vi "Return Devices with Forecasts.vi"(8 "Bus by ID":T2[](array[typedef]), 9 "ForecastData_Long":variant, 10 "DER_Info":variant, 11 "Generic Optimization in":refnum<class "Generic Optimization.lvclass">) -> (1 "Device Buses":dbl[](array[numeric]), 2 "Forecasts with Devices":T4[](array[typedef]), 3 "dup Generic Optimization out":refnum<class "Generic Optimization.lvclass">, 5 "Devices with Empty Forecasts":T1[](array[typedef]))   [LabVIEW 2018, in "Generic Optimization Actor.lvlib" / "Generic Optimization.lvclass"]
uses:
  Generic Optimization.lvclass
  <vilib>/ORNL/CSEISMIC DDS/CSEISMIC DDS Base/Data Types/ForecastData_Data.ctl
  <vilib>/ORNL/CSEISMIC DDS/CSEISMIC DDS Base/Data Types/Controls/DeviceID.ctl
  <vilib>/ORNL/CSEISMIC DDS/CSEISMIC DDS Base/Data Types/DER_Info.ctl
  Optimization Controls/Bus by ID.ctl
  C:/Users/Administrator/Desktop/2018LabVIEW EMS/EMS Generic Actor/EMS Generic/EMS Generic.lvclass
  <vilib>/ORNL/CSEISMIC DDS/CSEISMIC DDS Base/Data Types/Controls/DeviceClass Selector.ctl
  <vilib>/ORNL/CSEISMIC DDS/CSEISMIC DDS Base/CSEISMIC DDS.lvclass
  EMS Generic Actor/EMS Generic/EMS Generic.lvclass
panel:
  out "Devices with Forecasts":T3[](array[typedef])
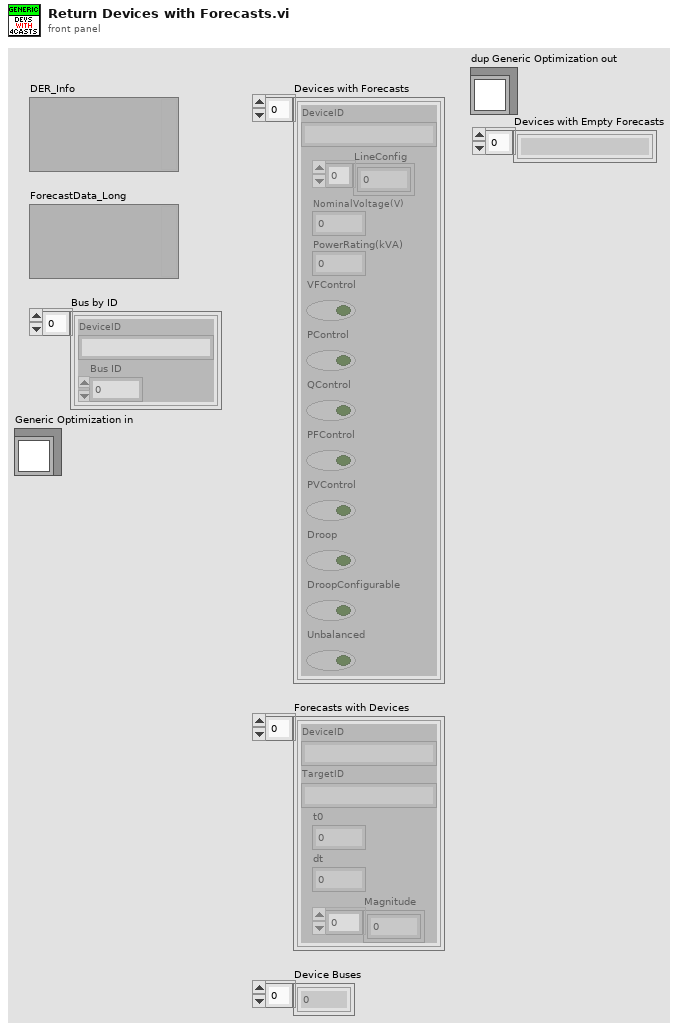
[diagram p1: front panel]
types:
  T1 = typedef "CSEISMIC DDS.lvlib/CSEISMIC DDS.lvclass/DeviceID.ctl" = string
  T2 = typedef "Generic Optimization Actor.lvlib/Generic Optimization.lvclass/Bus by ID.ctl" = cluster{"DeviceID":T1, "Bus ID":dbl}
  T3 = typedef "CSEISMIC DDS.lvlib/CSEISMIC DDS.lvclass/DER_Info.ctl" = cluster{"DeviceID":T1, "LineConfig":u8[], "NominalVoltage(V)":dbl, "PowerRating(kVA)":dbl, "VFControl":bool, "PControl":bool, "QControl":bool, "PFControl":bool, "PVControl":bool, "Droop":bool, "DroopConfigurable":bool, "Unbalanced":bool}
  T4 = typedef "CSEISMIC DDS.lvlib/CSEISMIC DDS.lvclass/ForecastData_Data.ctl" = cluster{"DeviceID":T1, "TargetID":T1, "t0":dbl, "dt":dbl, "Magnitude":dbl[]}
  T5 = typedef "CSEISMIC DDS.lvlib/CSEISMIC DDS.lvclass/DeviceClass Selector.ctl" = u16
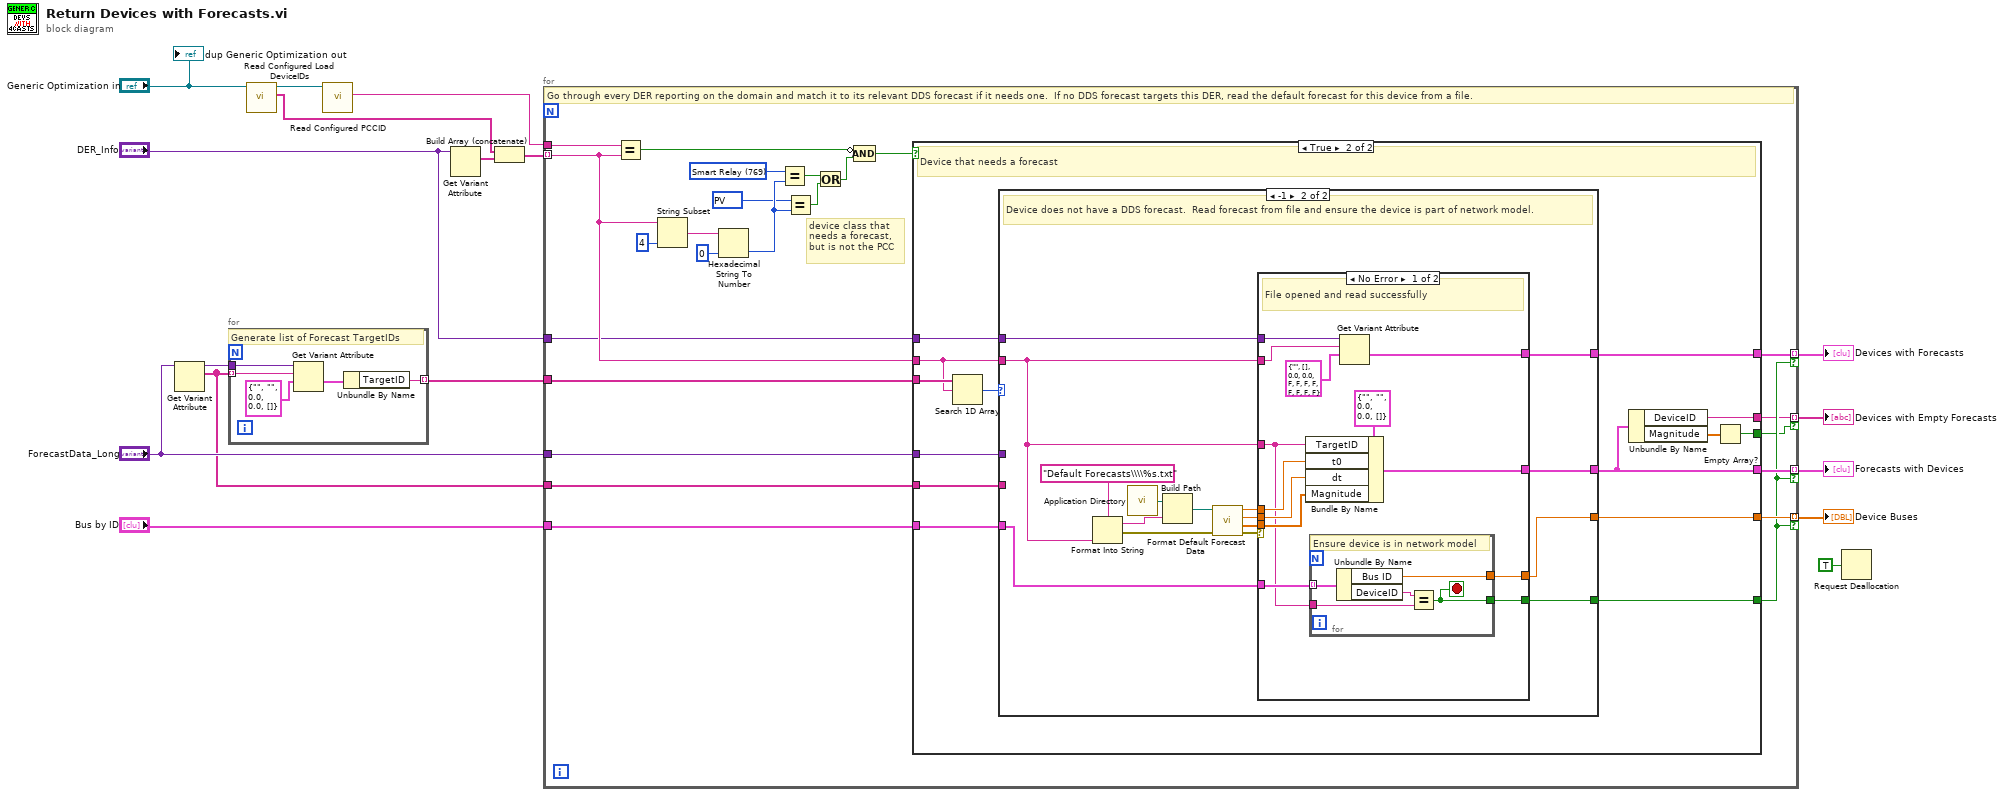
[diagram p0: block diagram]
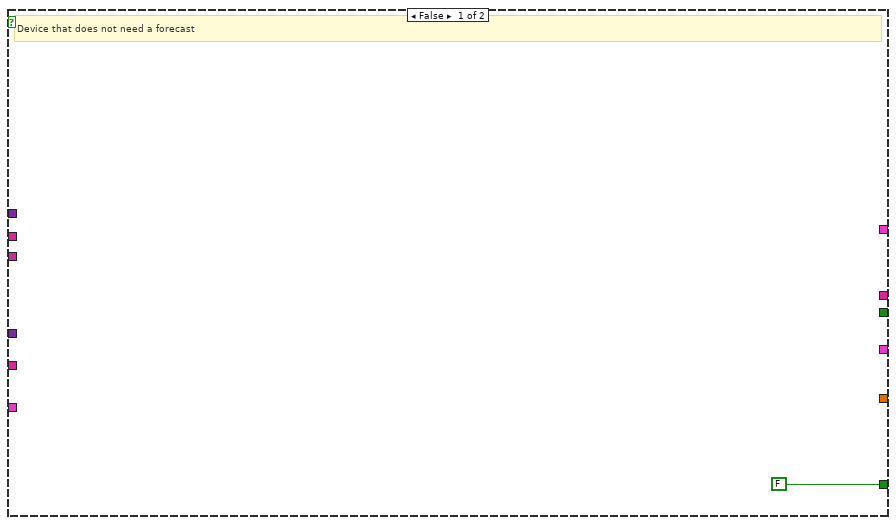
[diagram p2: hidden frame]
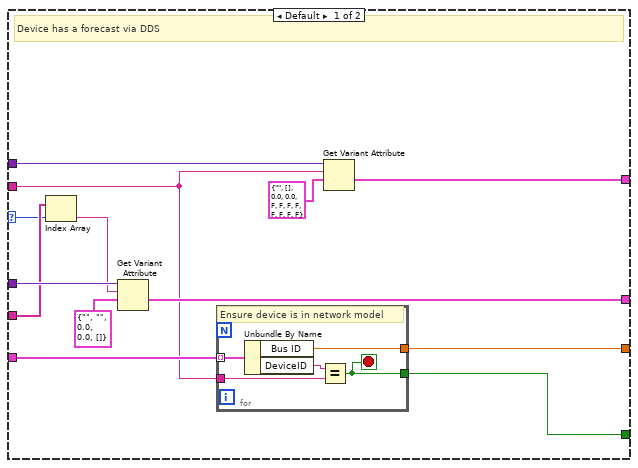
[diagram p3: hidden frame]
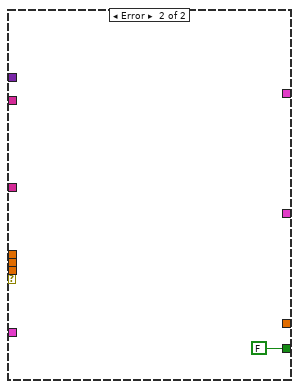
[diagram p4: hidden frame]
diagram:
  n1 = Get Variant Attribute(Variant="ForecastData_Long") -> (duplicate Variant=w11:variant, names=w8:string[])  [unwired: 3 in, 2 out]
  n2 = for {
    tunnel: w8 -> [w21] mode=indexing
    tunnel: w11 -> [w22]
    tunnel: [w18] -> w10 mode=indexing
    # "Generate list of Forecast TargetIDs"
    n3 = Get Variant Attribute(Variant=w22, name=w21, default value (empty Variant)=T4 {"DeviceID"="", "TargetID"="", "t0"=0.0, "dt"=0.0, "Magnitude"=[]} ("ForecastData")) -> (value=w19:T4)  [unwired: 1 in, 3 out]
    n4 = Unbundle By Name(w19) -> ("TargetID"=w18:T1)
  }
  n5 = call "Read Configured Load DeviceIDs.vi"("EMS Generic in"="Generic Optimization in") -> ("Load DeviceIDs"=w3:T1[], "EMS Generic out"=w5:refnum<class "Generic Optimization.lvclass">)  [unwired: 8 in, 1 out]
  n6 = call "Read Configured PCCID.vi"("EMS Generic in"=w5) -> ("PCCID"=w12:T1)  [unwired: 8 in, 2 out]
  n7 = Get Variant Attribute(Variant="DER_Info") -> (names=w4:string[])  [unwired: 3 in, 3 out]
  n8 = Build Array (concatenate)(w3, w4) -> (w7:T1[])
  n9 = for {
    tunnel: w7 -> [w34] mode=indexing
    tunnel: w12 -> [w36]
    tunnel: w10 -> [w33]
    tunnel: "Bus by ID" -> [w32]
    tunnel: "ForecastData_Long" -> [w31]
    tunnel: w8 -> [w30]
    tunnel: "DER_Info" -> [w29]
    tunnel: [w28] -> w13 mode=indexing if=w25
    tunnel: [w27] -> w17 mode=indexing if=w25
    tunnel: [w26] -> w16 mode=indexing if=w25
    tunnel: [w24] -> w1 mode=indexing if=w23
    w42 = T5 769 items=["Invalid"=0, "IED"=256, "DER"=512, "Relay"=768, "Meter"=1024, "Load"=1280, "Forecast"=1536, "Price"=1792, "Energy Storage"=513, "PV"=514, "Generator"=515, "Smart Relay"=769, "PCC"=770, "Smart Meter"=1025, "PMU"=1026, "HVAC"=1281] ("DeviceClass")
    w40 = T5 514 items=["Invalid"=0, "IED"=256, "DER"=512, "Relay"=768, "Meter"=1024, "Load"=1280, "Forecast"=1536, "Price"=1792, "Energy Storage"=513, "PV"=514, "Generator"=515, "Smart Relay"=769, "PCC"=770, "Smart Meter"=1025, "PMU"=1026, "HVAC"=1281] ("DeviceClass")
    # "device class that needs a forecast, but is not the PCC"
    # "Go through every DER reporting on the domain and match it to its relevant DDS forecast if it needs one.  If no DDS forecast targets this DER, read the default forecast for this device from a file."
    n10 = Equal?(x=w36, y=w34) -> (x = y?=w46:bool)
    n11 = String Subset(string=w34, length (rest)=4 ("length (rest)")) -> (substring=w38:T1)  [unwired: 1 in]
    n12 = Hexadecimal String To Number(string=w38, default (0uL)=u16 0 ("default (0 U32)")) -> (number=w41:u16)  [unwired: 1 in, 1 out]
    n13 = Equal?(x=w42, y=w41) -> (x = y?=w43:bool)
    n14 = Equal?(x=w40, y=w41) -> (x = y?=w44:bool)
    n15 = Or(x=w43, y=w44) -> (x .or. y?=w45:bool)
    n16 = Compound Arithmetic op=AND(invert w46, w45) -> (w35:bool)
    n17 = case shown="True" w35 {
      tunnel: w34 -> [_ w55]
      tunnel: w33 -> [_ w61]
      tunnel: w32 -> [_ w59]
      tunnel: w31 -> [_ w58]
      tunnel: w30 -> [_ w57]
      tunnel: w29 -> [_ w56]
      tunnel: [FALSE w54] -> w25
      tunnel: [_ w51] -> w27
      tunnel: [_ w53] -> w26
      tunnel: [_ w52] -> w28
      tunnel: [_ w50] -> w24
      tunnel: [_ w48] -> w23
      frame False {
        # "Device that does not need a forecast"
      }
      frame True {
        # "Device that needs a forecast"
        n18 = Search 1D Array(1D array=w61, element=w55) -> (index of element=w60:i32)  [unwired: 1 in]
        n19 = case shown="-1" w60 {
          selector: w60 -> [w65 _]
          tunnel: w59 -> [w74 w84]
          tunnel: w58 -> [w73 _]
          tunnel: w57 -> [w66 _]
          tunnel: w56 -> [w72 w85]
          tunnel: w55 -> [w62 w86]
          tunnel: [w71 w83] -> w52
          tunnel: [w70 w82] -> w51
          tunnel: [w69 w81] -> w53
          tunnel: [w68 w80] -> w54
          frame Default {
            # "Device has a forecast via DDS"
            n20 = Index Array(array=w66, index=w65) -> (element=w64:string)
            n21 = Get Variant Attribute(Variant=w73, name=w64, default value (empty Variant)=T4 {"DeviceID"="", "TargetID"="", "t0"=0.0, "dt"=0.0, "Magnitude"=[]} ("ForecastData")) -> (value=w70:T4)  [unwired: 1 in, 3 out]
            n22 = for {
              tunnel: w74 -> [w79] mode=indexing
              tunnel: w62 -> [w78]
              tunnel: [w76] -> w69
              tunnel: [w75] -> w68
              stop <- w75 stop-if-true
              # "Ensure device is in network model"
              n23 = Unbundle By Name(w79) -> ("Bus ID"=w76:dbl, "DeviceID"=w77:T1)
              n24 = Equal?(x=w77, y=w78) -> (x = y?=w75:bool)
            }
            n25 = Get Variant Attribute(Variant=w72, name=w62, default value (empty Variant)=T3 {"DeviceID"="", "LineConfig"=[], "NominalVoltage(V)"=0.0, "PowerRating(kVA)"=0.0, "VFControl"=FALSE, "PControl"=FALSE, "QControl"=FALSE, "PFControl"=FALSE, "PVControl"=FALSE, "Droop"=FALSE, "DroopConfigurable"=FALSE, "Unbalanced"=FALSE} ("DER_Info")) -> (value=w71:T3)  [unwired: 1 in, 3 out]
          }
          frame -1 {
            # "Device does not have a DDS forecast.  Read forecast from file and ensure the device is part of network model."
            n26 = Format Into String(format string="Default Forecasts\\\\%s.txt", w86) -> (resulting string=w93:string, error out=w92:errorcluster)  [unwired: 2 in]
            n27 = call <vilib>:"Application Directory.vi"() -> ("Application Directory"=w95:path)
            n28 = Build Path(base path=w95, name or relative path=w93) -> (appended path=w91:path)
            n29 = call "Format Default Forecast Data.vi"("error in"=w92, "file path"=w91) -> ("error out"=w87:errorcluster, "Data"=w88:dbl[], "dt (sec)"=w89:dbl, "t0 (sec)"=w90:dbl)  [unwired: 6 in]
            n30 = case shown="No Error" w87 {
              tunnel: w90 -> [w108 _]
              tunnel: w89 -> [w107 _]
              tunnel: w88 -> [w106 _]
              tunnel: [w105 _] -> w82
              tunnel: [w97 FALSE] -> w80
              tunnel: w86 -> [w98 _]
              tunnel: w86 -> [w102 _]
              tunnel: w85 -> [w103 _]
              tunnel: [w100 _] -> w83
              tunnel: w84 -> [w99 _]
              tunnel: [w96 _] -> w81
              frame No Error {
                # "File opened and read successfully"
                n31 = Bundle By Name(cluster=T4 {"DeviceID"="", "TargetID"="", "t0"=0.0, "dt"=0.0, "Magnitude"=[]} ("ForecastData"), "TargetID"=w98, "t0"=w108, "dt"=w107, "Magnitude"=w106) -> (w105:T4)
                n32 = for {
                  tunnel: w99 -> [w113] mode=indexing
                  tunnel: w98 -> [w112]
                  tunnel: [w110] -> w96
                  tunnel: [w109] -> w97
                  stop <- w109 stop-if-true
                  # "Ensure device is in network model"
                  n33 = Unbundle By Name(w113) -> ("Bus ID"=w110:dbl, "DeviceID"=w111:T1)
                  n34 = Equal?(x=w111, y=w112) -> (x = y?=w109:bool)
                }
                n35 = Get Variant Attribute(Variant=w103, name=w102, default value (empty Variant)=T3 {"DeviceID"="", "LineConfig"=[], "NominalVoltage(V)"=0.0, "PowerRating(kVA)"=0.0, "VFControl"=FALSE, "PControl"=FALSE, "QControl"=FALSE, "PFControl"=FALSE, "PVControl"=FALSE, "Droop"=FALSE, "DroopConfigurable"=FALSE, "Unbalanced"=FALSE} ("DER_Info")) -> (value=w100:T3)  [unwired: 1 in, 3 out]
              }
              frame Error {
              }
            }
          }
        }
        n36 = Unbundle By Name(w51) -> ("DeviceID"=w50:T1, "Magnitude"=w49:dbl[])
        n37 = Empty Array?(array=w49) -> (empty?=w48:bool)
      }
    }
  }
  "Forecasts with Devices" <- w17
  "Devices with Forecasts" <- w13
  "Device Buses" <- w16
  "Devices with Empty Forecasts" <- w1
  n38 = Request Deallocation(TRUE ("flag")) -> ()
  "dup Generic Optimization out" <- "Generic Optimization in"
